vi "SBG_Ellipse_check_length_n_end (SubVI).vi"(10 "x":i32, 11 "input String":string) -> (0 "length (debug)":i32, 2 "substring (debug)":string, 3 "is data ok?":bool)   [LabVIEW 2017]
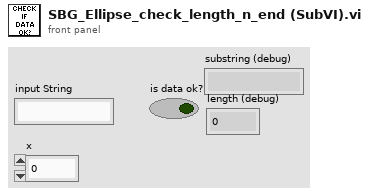
[diagram p1: front panel]
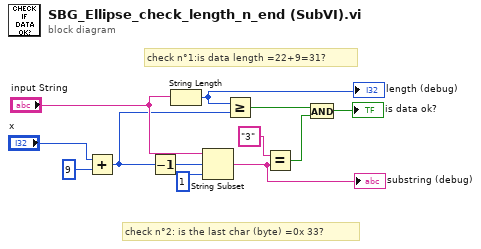
[diagram p0: block diagram]
diagram:
  # "check n°1:is data length =22+9=31?"
  # "check n°2: is the last char (byte) =0x 33?"
  n1 = Add(x="x", y=9) -> (x+y=w1:i32)
  n2 = Decrement(x=w1) -> (x-1=w9:i32)
  n3 = String Length(string="input String") -> (length=w2:i32)
  "length (debug)" <- w2
  n4 = String Subset(string="input String", offset (0)=w9, length (rest)=1 ("length (rest)")) -> (substring=w8:string)
  "substring (debug)" <- w8
  n5 = Greater Or Equal?(x=w2, y=w1) -> (x >= y?=w10:bool)
  n6 = Equal?(x="3", y=w8) -> (x = y?=w11:bool)
  n7 = And(x=w10, y=w11) -> (x .and. y?=→"is data ok?":bool)
